vi "Update Status Message for Test.vi"(11 "LCM1 Power On in":refnum<class "LCM1 Power On.lvclass">) -> ()   [LabVIEW 2015, in "LCM1 Power On.lvclass"]
uses:
  LCM1 Power On.lvclass
  Test Class/Test Class.lvclass
  Classes/Application/Class/Application.lvclass
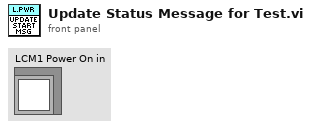
[diagram p1: front panel]
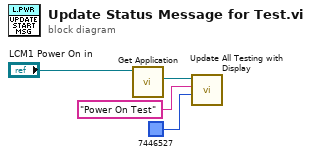
[diagram p0: block diagram]
diagram:
  n1 = call "Get Application.vi"("Test Class in"="LCM1 Power On in") -> ("Application.lvlib:Application.lvclass"=w4:refnum<class "Application.lvclass">)  [unwired: 9 in, 1 out]
  n2 = call "Update All Testing with Display.vi"("BG Color"=u32 7446527, "Message ('')"="Power On Test", "Application in"=w4) -> ()  [unwired: 7 in, 2 out]
